vi "Update-available-actions.vi"(8 "error in (no error)":errorcluster, 11 "Object ref in":T1) -> (0 "error out":errorcluster, 3 "Object ref out":T1)   [LabVIEW 2013, in "PowderDeposition.lvlib" / "PD-Main.lvclass"]
uses:
  PD-Main.lvclass
  Object-reference.ctl
  PD-Main.lvclass/PD-Main.ctl
  Motor/Motor.lvclass
  Assembly/Motor-assembly.lvclass
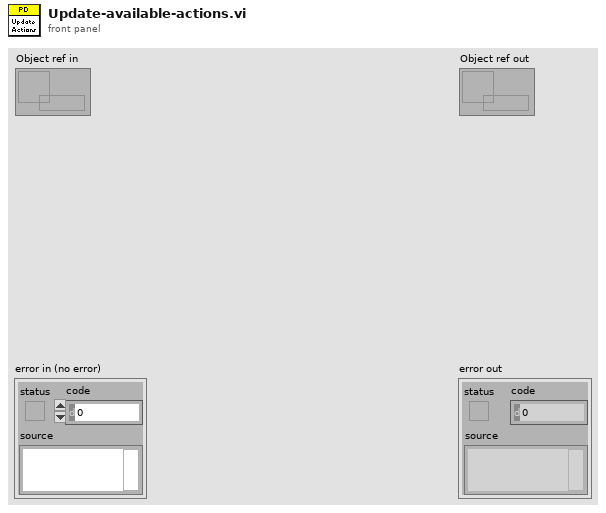
[diagram p1: front panel]
types:
  T1 = typedef "PowderDeposition.lvlib/PD-Main.lvclass/Object-reference.ctl" = refnum<data-value>
  T2 = typedef "PowderDeposition.lvlib/Action.lvclass/Motor-actions.ctl" = enum16{"Move - Absolute", "Move - Relative", "Move - Timer", "Wait", "Home", "Substrate", "Sieve", "Stop"}
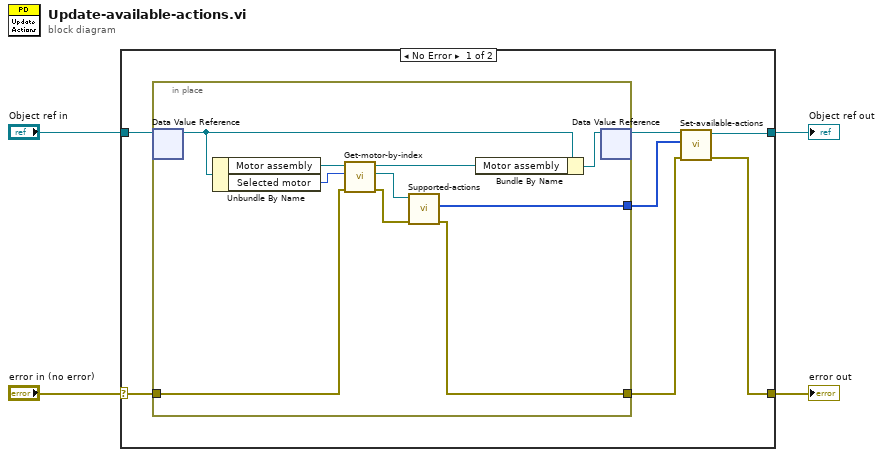
[diagram p0: block diagram]
diagram:
  n1 = case shown="No Error" "error in (no error)" {
    selector: "error in (no error)" -> [w10 w23]
    tunnel: [w5 w23] -> w3
    tunnel: [w6 w22] -> w1
    tunnel: "Object ref in" -> [w11 w22]
    frame No Error {
      n2 = in-place {
        in-place-border: [w12] -> w8
        in-place-border: w10 -> [w16]
        in-place-border: [w13] -> w7
        n3 = in-place-dvr #1(w11) -> (w21:refnum<class "PD-Main.lvclass">)  [unwired: 1 out]
        n4 = Unbundle By Name(w21) -> ("Motor assembly"=w18:refnum<class "Motor-assembly.lvclass">, "Selected motor"=w19:i32)
        n5 = call "Get-motor-by-index.vi"("error in (no error)"=w16, "Index"=w19, "Available motors in"=w18) -> ("error out"=w15:errorcluster, "Motor"=w14:refnum<class "Motor.lvclass">, "Available motors out"=w17:refnum<class "Motor-assembly.lvclass">)  [unwired: 5 in, 1 out]
        n6 = call-dynamic "Supported-actions.vi"("error in (no error)"=w15, "Motor in"=w14) -> ("error out"=w12:errorcluster, "Supported actions"=w13:T2[])  [unwired: 6 in, 2 out]
        n7 = Bundle By Name(cluster=w21, "Motor assembly"=w17) -> (w20:refnum<class "PD-Main.lvclass">)
        n8 = in-place-dvr #1(w20) -> (w9:T1)  [unwired: 1 out]
      }
      n9 = call "Set-available-actions.vi"("error in (no error)"=w8, "Supported actions"=w7, "Data in"=w9) -> ("error out"=w5:errorcluster, "Data out"=w6:T1)  [unwired: 7 in]
    }
    frame Error {
    }
  }
  "error out" <- w3
  "Object ref out" <- w1
